vi "FPGA_Main_R1.vi"() -> ()   [LabVIEW 2018]
uses:
  <vilib>/rvi/Emulation/niFpgaGetClockAttributes.vi
  <vilib>/rvi/Emulation/niFpgaSctlEmulationGetInTimedLoop.vi
  <vilib>/rvi/Emulation/niFpgaEmulationReportErrorSimple.vi
  <vilib>/IEDriver/SPIandI2C/FPGA/Private/Initialize Port (I2C).vi
  <vilib>/IEDriver/SPIandI2C/FPGA/Private/Configure Port (I2C).vi
  <vilib>/IEDriver/SPIandI2C/FPGA/Private/Read Port (I2C).vi
  <vilib>/IEDriver/SPIandI2C/FPGA/Private/Arm Port (I2C).vi
  <vilib>/IEDriver/SPIandI2C/FPGA/Private/Write Port (I2C).vi
  <vilib>/rvi/Emulation/niFpgaProcessEmulError.vi
  <vilib>/rvi/Emulation/niFpgaCriticalErrorInLSC.vi
  <vilib>/IEDriver/SPIandI2C/FPGA/Private/IP Port (I2C).vi
  <vilib>/IEDriver/SPIandI2C/FPGA/Library/IP SPI&I2C.lvlib
panel:
  out "Done":bool
  in  "Command Data":T1 {"Command (Write & Read)" items=["Write & Read", "Write", "Read"]}
  out "I2C Protocol State":T2(ring)
  out "Actual Rate (Hz)":u32
  in  "I2C Protocol Action":T2(ring)=enum."Idle"
  in  "I2C Protocol Input Data":u8
  out "I2C Protocol Output Data":u8
  in  "I2C Protocol Configure In":T3
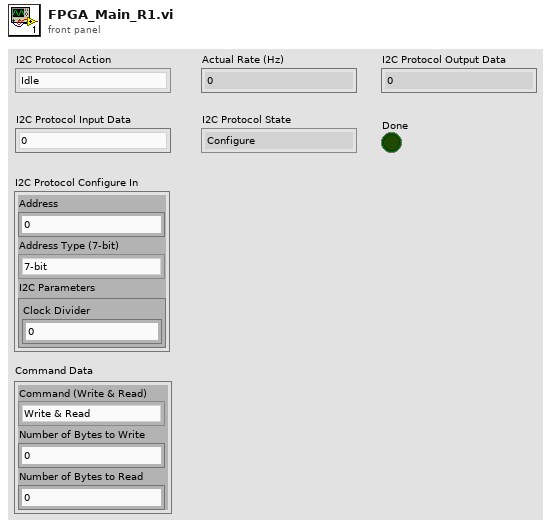
[diagram p1: front panel]
types:
  T1 = cluster{"Command (Write & Read)":u8, "Number of Bytes to Write":u16, "Number of Bytes to Read":u16}
  T2 = enum8{"Configure", "Write", "Arm", "Read", "Set Idle", "Idle"}
  T3 = cluster{"Address":u16, "Address Type (7-bit)":enum16{"7-bit", "10-bit"}, "I2C Parameters":cluster{"Clock Divider":u32}}
  T4 = typedef "IP SPI&I2C.lvlib/Private Data (I2C).ctl" = cluster{"Arm Trigger":refnum<k21>, "API to IP Data":refnum<k21>, "IP to API Data":refnum<k21>, "Configuration Register":refnum<k21>, "Configuration Lock":refnum<k21>}
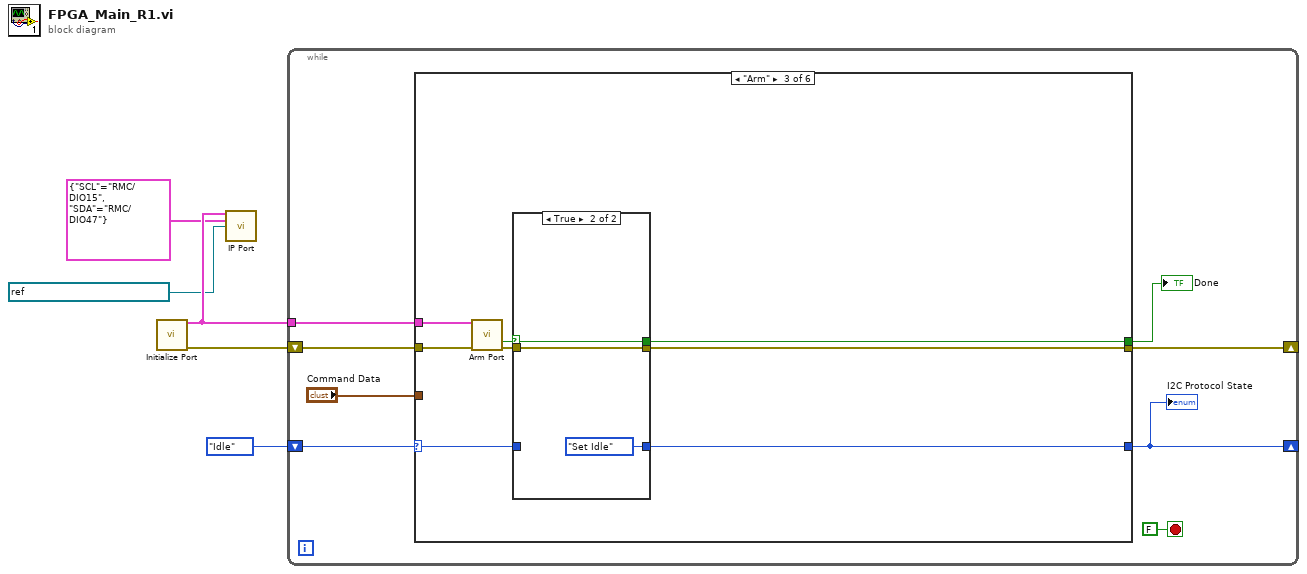
[diagram p0: block diagram]
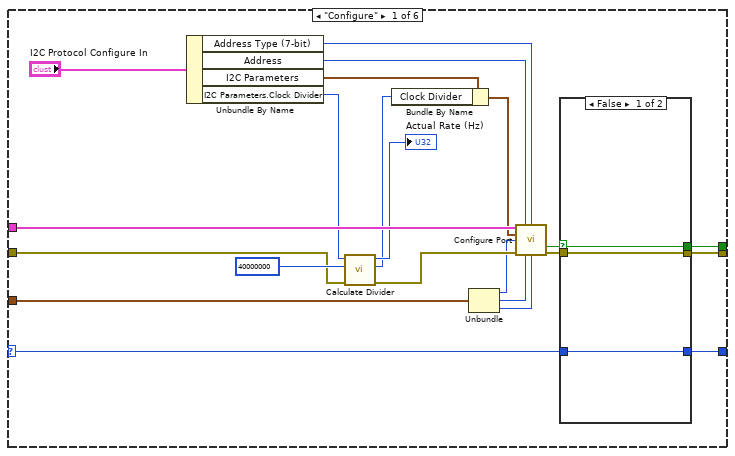
[diagram p2: hidden frame]
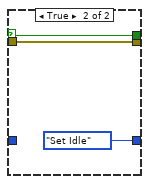
[diagram p3: hidden frame]
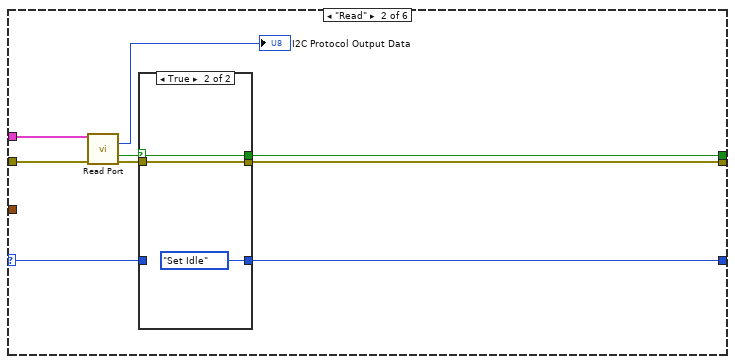
[diagram p4: hidden frame]
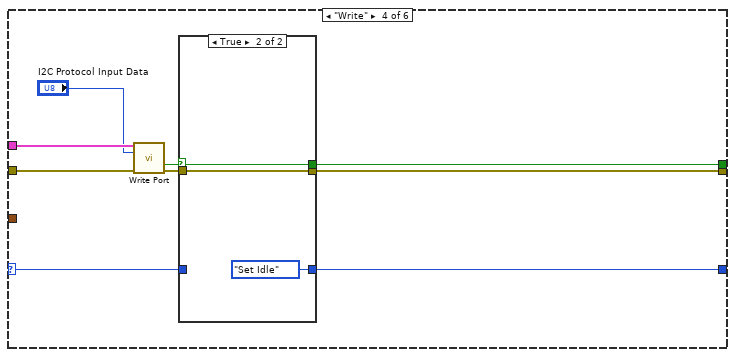
[diagram p7: hidden frame]
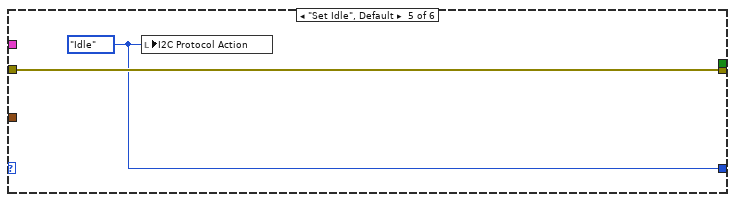
[diagram p9: hidden frame]
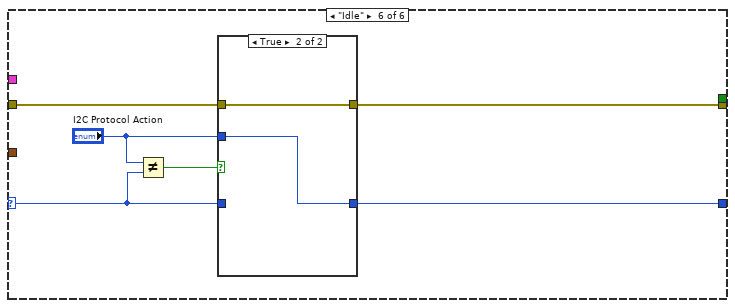
[diagram p10: hidden frame]
diagram:
  n1 = call-poly <vilib>:"Initialize Port.vi"() -> ("Private Data Out"=w4:T4, "error out"=w5:errorcluster)  [unwired: 14 in]
  n2 = call-poly <vilib>:"IP Port.vi"("Private Data In"=w4, "I2C FPGA IO"=cluster{"SCL":refnum<k21>, "SDA":refnum<k21>} {"SCL"="RMC/DIO15", "SDA"="RMC/DIO47"}, "FPGA Clock"=refnum<k21> "40 MHz Onboard Clock") -> ()  [unwired: 13 in]
  n3 = while {
    shift-right: [w8] -> _
    shift-left: w5 -> [w12]
    tunnel: w4 -> [w13]
    shift-right: [w9] -> _
    shift-left: T2."Idle" ("Action") -> [w10]
    stop <- FALSE stop-if-true
    n4 = case shown="\"Arm\"" w10 {
      selector: w10 -> [w26 w46 w60 w74 _ w90]
      tunnel: w13 -> [w35 w50 w64 w79 _ _]
      tunnel: w12 -> [w33 w49 w63 w78 w87 w92]
      tunnel: [w27 w43 w58 w72 w87 w91] -> w8
      tunnel: [w25 w44 w59 w73 w86 w88] -> w9
      tunnel: "Command Data" -> [w24 _ _ _ _ _]
      tunnel: [w14 w42 w57 w71 _ _] -> w6
      frame "Configure" {
        n5 = Unbundle By Name("I2C Protocol Configure In") -> ("Address Type (7-bit)"=w23:enum16{"7-bit", "10-bit"}, "Address"=w22:u16, "I2C Parameters"=w20:cluster{"Clock Divider":u32}, "I2C Parameters.Clock Divider"=w21:u32)
        n6 = call <vilib>:"Calculate Divider.vi"("error in"=w33, "FPGA Clock (Hz)"=u32 40000000, "Clock Rate (Hz)"=w21) -> ("error out"=w30:errorcluster, "Clock Divider"=w19:u32, "Actual Rate (Hz)"=→"Actual Rate (Hz)":u32)  [unwired: 6 in]
        n7 = Bundle By Name(cluster=w20, "Clock Divider"=w19) -> (w18:cluster{"Clock Divider":u32})
        n8 = Unbundle(w24) -> ("Command (Write & Read)"=w17:u8, "Number of Bytes to Write"=w16:u16, "Number of Bytes to Read"=w15:u16)
        n9 = call-poly <vilib>:"Configure Port.vi"("Private Data In"=w35, "Address"=w22, "Address Type (7-bit)"=w23, "I2C Parameters"=w18, "Command (Write & Read)"=w17, "error in"=w30, "Number of Bytes to Write"=w16, "Number of Bytes to Read"=w15) -> ("Done"=w29:bool, "error out"=w28:errorcluster)  [unwired: 5 in, 1 out]
        n10 = case shown="False" w29 {
          selector: w29 -> [w36 w39]
          tunnel: w28 -> [w38 w41]
          tunnel: [w38 w41] -> w27
          tunnel: w26 -> [w37 _]
          tunnel: [w37 T2."Set Idle" ("Action")] -> w25
          tunnel: [w36 w39] -> w14
          frame False {
          }
          frame True {
          }
        }
      }
      frame "Read" {
        n11 = call-poly <vilib>:"Read Port.vi"("Private Data In"=w50, "error in"=w49) -> ("Data Out"=→"I2C Protocol Output Data":u8, "Output Valid"=w47:bool, "error out"=w45:errorcluster)  [unwired: 10 in, 1 out]
        n12 = case shown="True" w47 {
          selector: w47 -> [w51 w54]
          tunnel: w46 -> [w53 _]
          tunnel: w45 -> [w52 w56]
          tunnel: [w53 T2."Set Idle" ("Action")] -> w44
          tunnel: [w52 w56] -> w43
          tunnel: [w51 w54] -> w42
          frame False {
          }
          frame True {
          }
        }
      }
      frame "Arm" {
        n13 = call-poly <vilib>:"Arm Port.vi"("Private Data In"=w64, "error in"=w63) -> ("Done"=w62:bool, "error out"=w61:errorcluster)  [unwired: 11 in, 1 out]
        n14 = case shown="True" w62 {
          selector: w62 -> [w65 w68]
          tunnel: w61 -> [w66 w69]
          tunnel: w60 -> [w67 _]
          tunnel: [w67 T2."Set Idle" ("Action")] -> w59
          tunnel: [w66 w69] -> w58
          tunnel: [w65 w68] -> w57
          frame False {
          }
          frame True {
          }
        }
      }
      frame "Write" {
        n15 = call-poly <vilib>:"Write Port.vi"("Private Data In"=w79, "Data In"="I2C Protocol Input Data", "error in"=w78) -> ("Done"=w75:bool, "error out"=w76:errorcluster)  [unwired: 10 in, 1 out]
        n16 = case shown="True" w75 {
          selector: w75 -> [w80 w83]
          tunnel: w76 -> [w81 w84]
          tunnel: w74 -> [w82 _]
          tunnel: [w82 T2."Set Idle" ("Action")] -> w73
          tunnel: [w81 w84] -> w72
          tunnel: [w80 w83] -> w71
          frame False {
          }
          frame True {
          }
        }
      }
      frame "Set Idle", Default {
        w86 = T2."Idle" ("Action")
        n17 = local write "I2C Protocol Action"(w86) -> ()
      }
      frame "Idle" {
        n18 = Not Equal?(x="I2C Protocol Action", y=w90) -> (x != y?=w93:bool)
        n19 = case shown="True" w93 {
          tunnel: w92 -> [w95 w97]
          tunnel: [w95 w97] -> w91
          tunnel: w90 -> [w94 _]
          tunnel: "I2C Protocol Action" -> [_ w96]
          tunnel: [w94 w96] -> w88
          frame False {
          }
          frame True {
          }
        }
      }
    }
    "I2C Protocol State" <- w9
    "Done" <- w6
  }
